vi "Send Audio Out (SubVI)- 4 track.vi"(8 "error in (no error)":errorcluster, 10 "4-Track Audio out":T1, 11 "Refnum in":T3) -> (0 "error out":errorcluster, 3 "Refnum out":T3)   [LabVIEW 2014]
uses:
  Controls/FPGA Reference.ctl
  Controls/4 Track Audio.ctl
  Controls/Audio In.ctl
  <vilib>/Utility/error.llb/Error Cluster From Error Code.vi
  <vilib>/rvi/errors/niLvFpgaAdjustHostInterfaceError.vi
  <vilib>/rvi/interface/nirviMethod/nirviMethod.xnode
  <vilib>/FPGAPlugInAG/Dynamic/niLvFpga_WriteFifo_Dynamic.vi
  <vilib>/rvi/errors/niLvFpgaMergeErrorWithErrorCode.vi
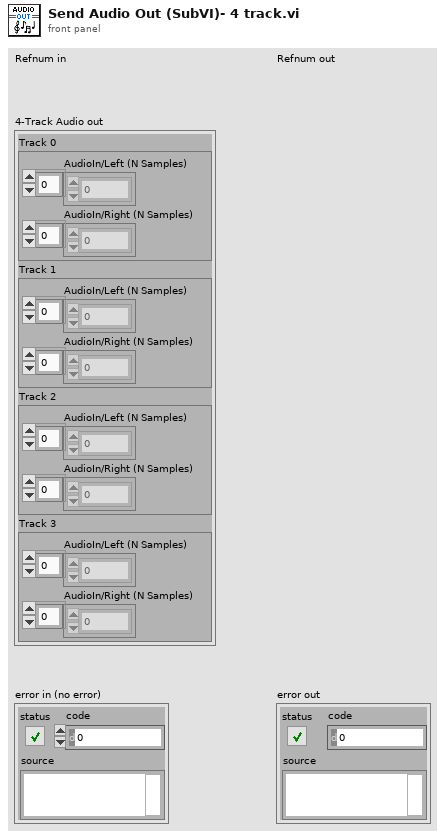
[diagram p1: front panel]
types:
  T1 = typedef "4 Track Audio.ctl" = cluster{"Track 0":T2, "Track 1":T2, "Track 2":T2, "Track 3":T2}
  T2 = typedef "Audio In.ctl" = cluster{"AudioIn/Left (N Samples)":i16[], "AudioIn/Right (N Samples)":i16[]}
  T3 = typedef "FPGA Reference.ctl" = refnum<k20>
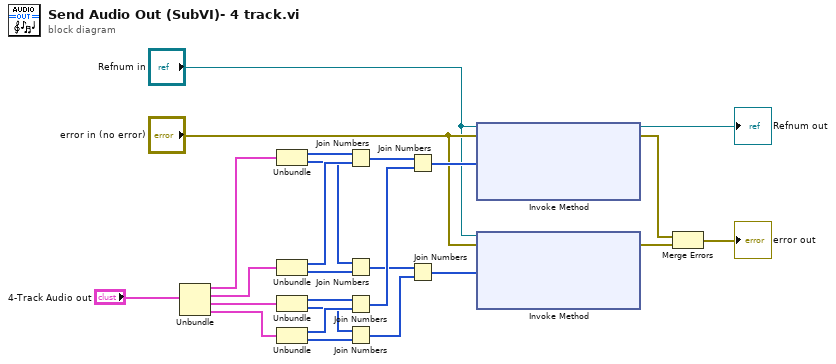
[diagram p0: block diagram]
diagram:
  n1 = Unbundle("4-Track Audio out") -> ("Track 0"=w23:T2, "Track 1"=w22:T2, "Track 2"=w21:T2, "Track 3"=w20:T2)
  n2 = Unbundle(w23) -> ("AudioIn/Left (N Samples)"=w19:i16[], "AudioIn/Right (N Samples)"=w13:i16[])
  n3 = Unbundle(w22) -> ("AudioIn/Left (N Samples)"=w18:i16[], "AudioIn/Right (N Samples)"=w12:i16[])
  n4 = Unbundle(w21) -> ("AudioIn/Left (N Samples)"=w17:i16[], "AudioIn/Right (N Samples)"=w11:i16[])
  n5 = Unbundle(w20) -> ("AudioIn/Left (N Samples)"=w16:i16[], "AudioIn/Right (N Samples)"=w10:i16[])
  n6 = Join Numbers(hi=w19, lo=w18) -> ((hi.lo)=w15:u32[])
  n7 = Join Numbers(hi=w13, lo=w12) -> ((hi.lo)=w9:u32[])
  n8 = Join Numbers(hi=w17, lo=w16) -> ((hi.lo)=w14:u32[])
  n9 = Join Numbers(hi=w11, lo=w10) -> ((hi.lo)=w8:u32[])
  n10 = Join Numbers(hi=w15, lo=w14) -> ((hi.lo)=w7:u64[])
  n11 = Join Numbers(hi=w9, lo=w8) -> ((hi.lo)=w1:u64[])
  n12 = xnode "Invoke Method"("FPGA VI Reference In"="Refnum in", "error in"="error in (no error)", "Data"=w7) -> ("FPGA VI Reference Out"=→"Refnum out":T3, "error out"=w4:errorcluster)  [unwired: 1 in, 1 out]
  n13 = xnode "Invoke Method"("FPGA VI Reference In"="Refnum in", "error in"="error in (no error)", "Data"=w1) -> ("error out"=w3:errorcluster)  [unwired: 1 in, 2 out]
  n14 = Merge Errors(w4, w3) -> (→"error out":errorcluster)
